vi "PIM Handle Swept Plot.vi"(4 "Clear Plot? (f)":bool, 5 "Hold? (f)":bool, 7 "IM Power":dbl format="%.2f", 8 "IM Freq":dbl format="%.2f", 9 "Sweep Sizes":i32[](array[numeric])) -> (0 "Sweep Done?":bool, 1 "Current Count":i32, 2 "F1 Up Trace":cluster{"new array":dbl[], "new array":dbl[]} {"new array" format="%.2f"; "new array" format="%.2f"}, 3 "F2 Down Trace":cluster{"new array":dbl[], "new array":dbl[]} {"new array" format="%.2f"; "new array" format="%.2f"})   [LabVIEW 2011]
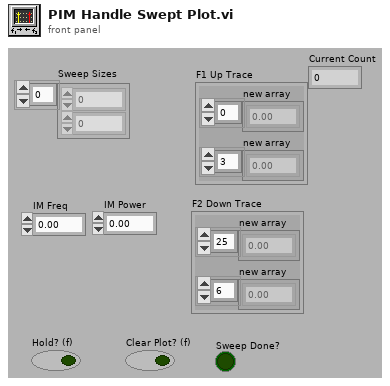
[diagram p1: front panel]
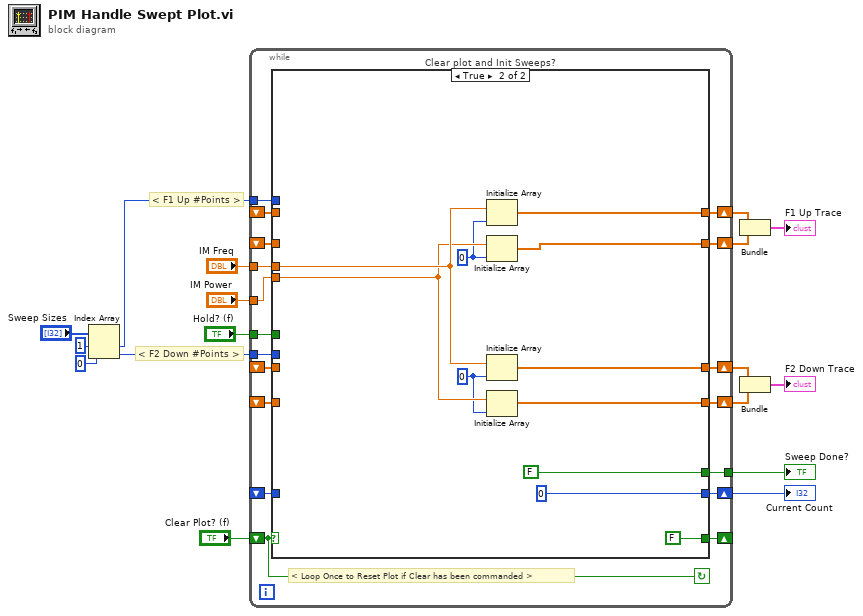
[diagram p0: block diagram]
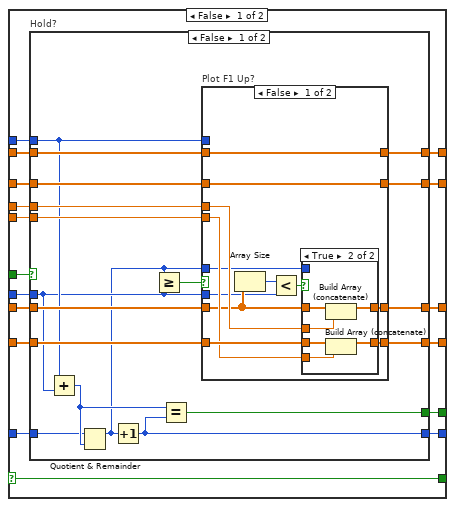
[diagram p2: hidden frame]
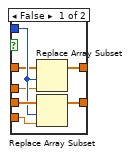
[diagram p3: hidden frame]
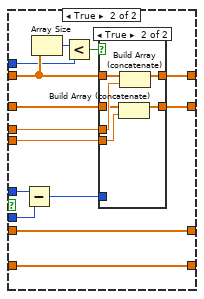
[diagram p4: hidden frame]
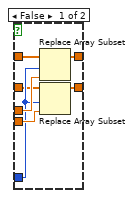
[diagram p5: hidden frame]
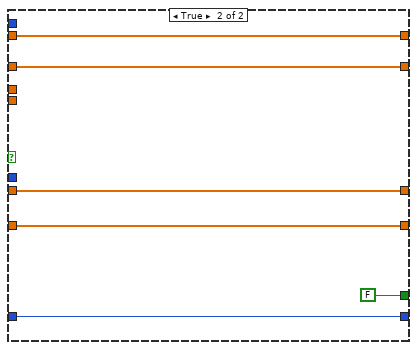
[diagram p6: hidden frame]
diagram:
  # "< F2 Down #Points >"
  # "< F1 Up #Points >"
  n1 = Index Array(array="Sweep Sizes", index #1=1 ("Index"), index #2=0) -> (element #1=w3:i32, element #2=w2:i32)
  n2 = while {
    tunnel: [w22] -> w10
    shift-left: _ -> [w25]
    shift-right: [w26] -> w11
    tunnel: "Hold? (f)" -> [w27]
    shift-left: _ -> [w29]
    shift-right: [w31] -> w12
    shift-left: _ -> [w30]
    shift-right: [w33] -> w7
    shift-left: _ -> [w28]
    shift-right: [w32] -> w13
    shift-left: _ -> [w24]
    shift-right: [w23] -> w1
    tunnel: "IM Freq" -> [w35]
    tunnel: "IM Power" -> [w34]
    tunnel: w3 -> [w21]
    tunnel: w2 -> [w20]
    shift-right: [w19] -> _
    shift-left: "Clear Plot? (f)" -> [w18]
    stop <- w18 continue-if-true
    # "< Loop Once to Reset Plot if Clear has been commanded >"
    n3 = case "Clear plot and Init Sweeps?" shown="True" w18 {
      selector: w18 -> [w36 _]
      tunnel: w35 -> [w47 w139]
      tunnel: w34 -> [w50 w138]
      tunnel: [w45 w135] -> w33
      tunnel: [w48 w136] -> w32
      tunnel: [w46 w134] -> w26
      tunnel: [w51 w137] -> w31
      tunnel: w30 -> [w44 _]
      tunnel: w29 -> [w52 _]
      tunnel: w28 -> [w49 _]
      tunnel: w27 -> [w43 _]
      tunnel: w25 -> [w42 _]
      tunnel: w24 -> [w41 _]
      tunnel: [w40 0] -> w23
      tunnel: [w39 FALSE] -> w22
      tunnel: w21 -> [w37 _]
      tunnel: w20 -> [w38 _]
      tunnel: [w36 FALSE] -> w19
      frame False {
        n4 = case "Hold?" shown="False" w43 {
          tunnel: w52 -> [w61 w128]
          tunnel: [w70 w128] -> w51
          tunnel: w50 -> [w69 _]
          tunnel: w49 -> [w68 w126]
          tunnel: [w67 w126] -> w48
          tunnel: w47 -> [w66 _]
          tunnel: [w65 w125] -> w46
          tunnel: [w64 w127] -> w45
          tunnel: w44 -> [w63 w127]
          tunnel: w42 -> [w62 w125]
          tunnel: w41 -> [w58 w124]
          tunnel: [w56 w124] -> w40
          tunnel: [w60 FALSE] -> w39
          tunnel: w38 -> [w54 _]
          tunnel: w37 -> [w57 _]
          frame False {
            n5 = Add(x=w57, y=w54) -> (x+y=w59:i32)
            n6 = Quotient & Remainder(x=w58, y=w59) -> (x-y*floor(x/y)=w53:i32)  [unwired: 1 out]
            n7 = Increment(x=w53) -> (x+1=w56:i32)
            n8 = Greater Or Equal?(x=w53, y=w54) -> (x >= y?=w55:bool)
            n9 = Equal?(x=w59, y=w56) -> (x = y?=w60:bool)
            n10 = case "Plot F1 Up?" shown="False" w55 {
              tunnel: w61 -> [w82 w103]
              tunnel: [w82 w109] -> w70
              tunnel: w69 -> [w79 w108]
              tunnel: w68 -> [w81 w107]
              tunnel: [w80 w107] -> w67
              tunnel: w53 -> [w71 w100]
              tunnel: w66 -> [w77 w106]
              tunnel: [w76 w105] -> w65
              tunnel: [w78 w104] -> w64
              tunnel: w63 -> [w75 w104]
              tunnel: w62 -> [w76 w102]
              tunnel: w54 -> [w73 w99]
              tunnel: w57 -> [_ w98]
              frame False {
                n11 = Array Size(array=w75) -> (size(s)=w72:i32)
                n12 = Less?(x=w72, y=w73) -> (x < y?=w74:bool)
                n13 = case shown="True" w74 {
                  tunnel: w81 -> [w89 w91]
                  tunnel: [w88 w92] -> w80
                  tunnel: w79 -> [w87 w90]
                  tunnel: w71 -> [w86 _]
                  tunnel: [w85 w94] -> w78
                  tunnel: w77 -> [w84 w93]
                  tunnel: w75 -> [w83 w95]
                  frame False {
                    n14 = Replace Array Subset(array=w83, new element=w84, index=w86) -> (w85:dbl[])
                    n15 = Replace Array Subset(array=w89, new element=w87, index=w86) -> (w88:dbl[])
                  }
                  frame True {
                    n16 = Build Array (concatenate)(w95, w93) -> (w94:dbl[])
                    n17 = Build Array (concatenate)(w91, w90) -> (w92:dbl[])
                  }
                }
              }
              frame True {
                n18 = Subtract(x=w100, y=w99) -> (x-y=w96:i32)
                n19 = Array Size(array=w102) -> (size(s)=w97:i32)
                n20 = Less?(x=w97, y=w98) -> (x < y?=w101:bool)
                n21 = case shown="True" w101 {
                  tunnel: [w116 w117] -> w109
                  tunnel: w108 -> [w115 w118]
                  tunnel: w106 -> [w114 w120]
                  tunnel: [w113 w121] -> w105
                  tunnel: w96 -> [w112 _]
                  tunnel: w102 -> [w111 w122]
                  tunnel: w103 -> [w110 w119]
                  frame False {
                    n22 = Replace Array Subset(array=w111, new element=w114, index=w112) -> (w113:dbl[])
                    n23 = Replace Array Subset(array=w110, new element=w115, index=w112) -> (w116:dbl[])
                  }
                  frame True {
                    n24 = Build Array (concatenate)(w119, w118) -> (w117:dbl[])
                    n25 = Build Array (concatenate)(w122, w120) -> (w121:dbl[])
                  }
                }
              }
            }
          }
          frame True {
          }
        }
      }
      frame True {
        w132 = 0 ("Dimension Size")
        w133 = 0 ("Dimension Size")
        n26 = Initialize Array(w139, w132) -> (w134:dbl[])
        n27 = Initialize Array(w138, w132) -> (w137:dbl[])
        n28 = Initialize Array(w139, w133) -> (w135:dbl[])
        n29 = Initialize Array(w138, w133) -> (w136:dbl[])
      }
    }
  }
  "Sweep Done?" <- w10
  "Current Count" <- w1
  n30 = Bundle(w11, w12) -> (→"F1 Up Trace":cluster{dbl[], dbl[]})  [unwired: 1 out]
  n31 = Bundle(w7, w13) -> (→"F2 Down Trace":cluster{dbl[], dbl[]})  [unwired: 1 out]
